vi "SR430_us_2_bin_width.vi"(2 "bin width [us]":dbl format="%.3f", 5 "error in (no error)":errorcluster) -> (16 "binWidth":i32, 17 "InRange?":bool, 19 "error out":errorcluster)   [LabVIEW 2009, in "SR430Driver.lvlib"]
doc: "converts the bin width in microseconds into the bin width in the format used by the units. Intermdiate values are rounded to the lower number.\n\nVI Tree for the SR430 Multi-Channel Scaler from Staford Research Systems.\n\nHistory: 24-APR-2002, Dietrich Beck\n\nCopyright (C)\nGesellschaft für Schwerionenforschung, GSI\nPlanckstr. 1\n64291 Darmstadt\nGermany\n\nContact: D.Beck@gsi.de \n\nThis program is free software; you can redistribute it and/or modify it under the terms of the \nGNU General Public License as published by the Free Software Foundation; either version 2 of the license, or (at your option) any later version.\n\nThis program is distributed in the hope that it will be useful, but WITHOUT ANY WARRANTY; without even the implied warranty of MERCHANTABILITY or FITNESS FOR A PARTICULAR PURPOSE. See the GNU General License for more details (http://www.gnu.org).\n\nGesellschaft für Schwerionenforschung, GSI\nPlanckstr. 1, 64291 Darmstadt, Germany\nFor all questions and ideas contact: M.Richter@gsi.de, K.Poppensieker, H.Brand@gsi.de or D.Beck@gsi.de.\nLast update: 11-APR-2002"
uses:
  SR430Driver.lvlib
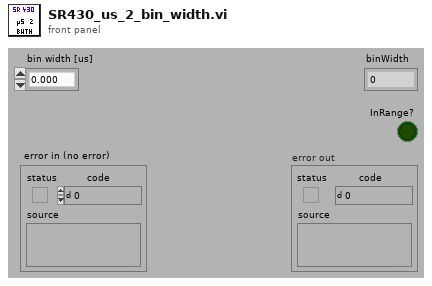
[diagram p1: front panel]
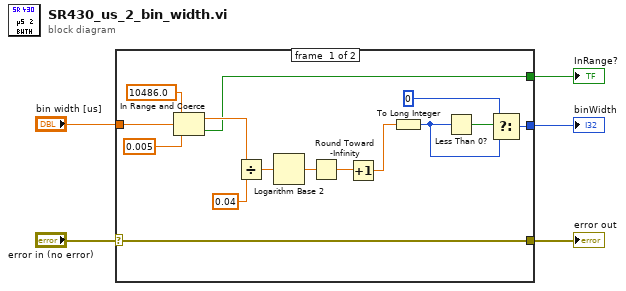
[diagram p0: block diagram]
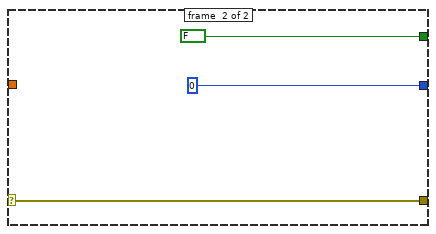
[diagram p2: hidden frame]
diagram:
  n1 = case shown="No Error" "error in (no error)" {
    selector: "error in (no error)" -> [w15 w23]
    tunnel: [w15 w23] -> w4
    tunnel: "bin width [us]" -> [w14 _]
    tunnel: [w9 0] -> w2
    tunnel: [w10 FALSE] -> w1
    frame #0 {
      n2 = In Range and Coerce(upper limit=10486.0, x=w14, lower limit=0.005) -> (coerced(x)=w11:dbl, In Range?=w10:bool)
      n3 = Divide(x=w11, y=0.04) -> (x/y=w17:dbl)
      n4 = Logarithm Base 2(1:w17) -> (0:w16:dbl)
      n5 = Round Toward -Infinity ("Round To -Infinity")(1:w16) -> (0:w19:dbl)
      n6 = Increment(x=w19) -> (x+1=w20:dbl)
      n7 = To Long Integer(number=w20) -> (32bit integer=w7:i32)
      n8 = Less Than 0?(x=w7) -> (x < 0?=w8:bool)
      n9 = Select(t=0, s=w8, f=w7) -> (s? t:f=w9:i32)
    }
    frame #1 {
    }
  }
  "error out" <- w4
  "binWidth" <- w2
  "InRange?" <- w1
